vi "Set Key To INI File.vi"(7 "keyValue":string, 8 "error in (no error)":errorcluster, 9 "keyName":string, 10 "sectionName":string, 11 "Sections in":refnum<k24>) -> (0 "error out":errorcluster, 3 "Sections out":refnum<k24>)   [LabVIEW 2015]
uses:
  C:/C-BOX/Utilities/dotNET/C-BOX/INIFileParser.dll
  C-BOX/Utilities/dotNET/C-BOX/INIFileParser.dll
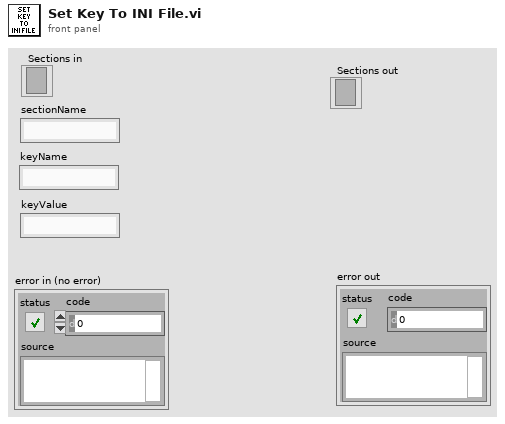
[diagram p1: front panel]
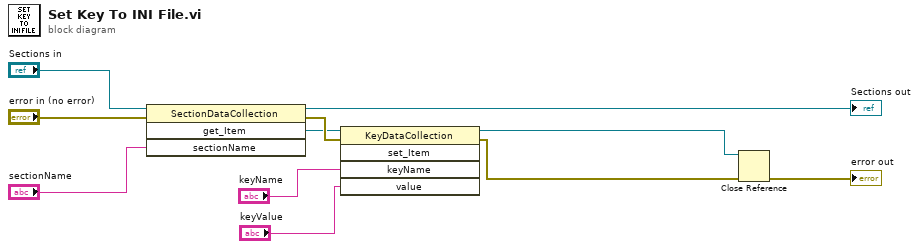
[diagram p0: block diagram]
diagram:
  n1 = invoke class="SectionDataCollection" method="get_Item"(reference="Sections in", error in="error in (no error)", "sectionName"="sectionName") -> (reference out=→"Sections out":refnum<k24>, error out=w11:errorcluster, "get_Item"=w10:refnum<k24>)  [unwired: 1 in, 1 out]
  n2 = invoke class="KeyDataCollection" method="set_Item"(reference=w10, error in=w11, "keyName"="keyName", "value"="keyValue") -> (reference out=w1:refnum<k24>, error out=w2:errorcluster)  [unwired: 1 in, 3 out]
  n3 = Close Reference(reference=w1, error in (no error)=w2) -> (error out=→"error out":errorcluster)
